vi "Read Test Data (DC Parallel Total Manual Mode).vi"(0 "VISA resource name":refnum<visa-resource-name>, 11 "error in (no error)":errorcluster) -> (4 "VISA resource name out":refnum<visa-resource-name>, 6 "Test Meter Data Output":T1 {"Voltage (V)" format="%.1f"; "RMS Current (A)" format="%.3f"; "Power (W)" format="%.1f"}, 15 "error out":errorcluster)   [LabVIEW 2016, in "APT 300XAC Series.lvlib"]
doc: "Reads the DC mode <B>active data being displayed on the LCD display</B> while the test is in process. It also gives the last data taken when the test sequence compled. \n\nIn DC Mode the output data cluster has the following data.\n\n1. Memory\n2. Timer (s)\n3. Voltage (V)\n4. RMS Current (A)\n5. Power (W)\n6. Status"
uses:
  APT 300XAC Series.lvlib
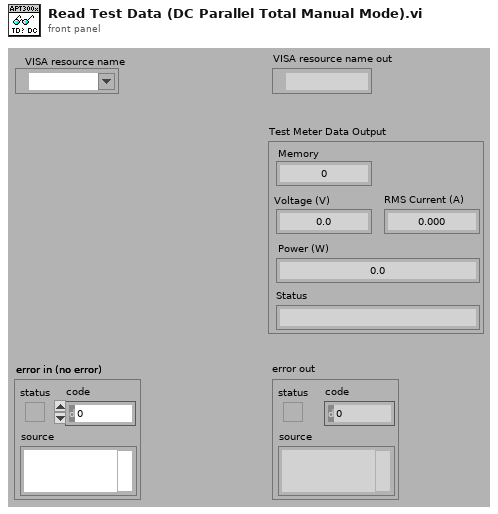
[diagram p1: front panel]
types:
  T1 = cluster{"Memory":dbl, "Voltage (V)":dbl, "RMS Current (A)":dbl, "Power (W)":dbl, "Status":string}
  T2 = cluster{"Memory":i32, "Volt":dbl, "Current":dbl, "Power":dbl, "Status":string}
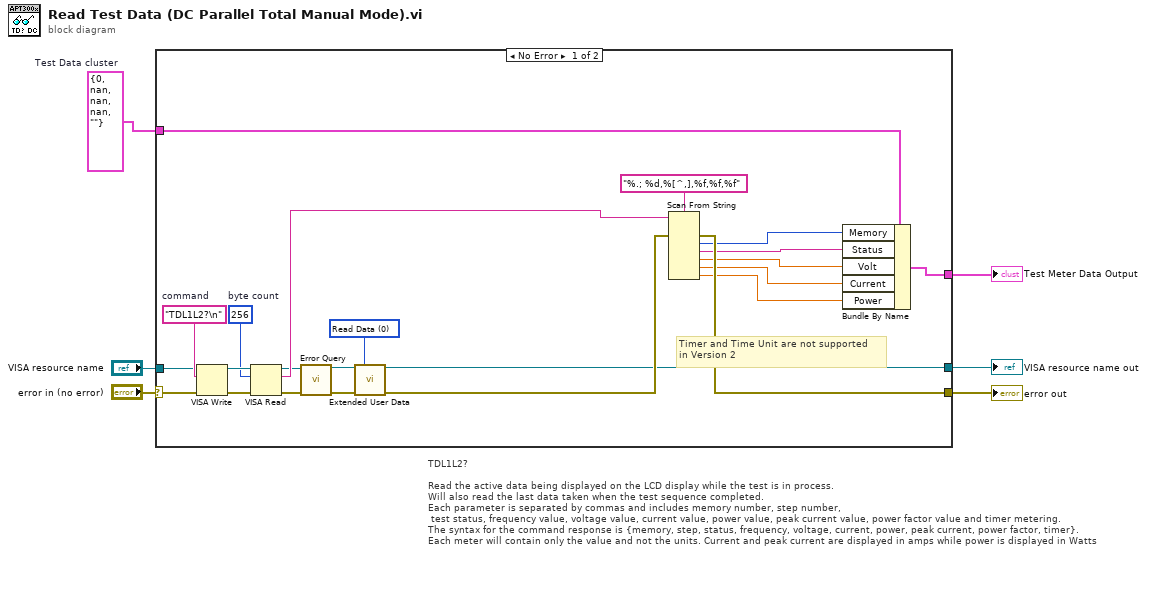
[diagram p0: block diagram]
diagram:
  w2 = T2 {"Memory"=0, "Volt"=nan, "Current"=nan, "Power"=nan, "Status"=""}  # Test Data cluster
  # "TDL1L2?\n\nRead the active data being displayed on the LCD display while the test is in process. \nWill also read the last data taken when the test sequence completed. \nEach parameter is separated by commas and includes memory number, step number,\n test status, frequency value, voltage value, current value, power value, peak current value, power factor value and timer metering. \nThe syntax for the command response is {memory, step, status, frequency, voltage, current, power, peak current, power factor, timer}. \nEach meter will contain only the value and not the units. Current and peak current are displayed in amps while power is displayed in Watts"
  n1 = case shown="No Error" "error in (no error)" {
    selector: "error in (no error)" -> [w22 w31]
    tunnel: "VISA resource name" -> [w23 w32]
    tunnel: [w13 w32] -> w4
    tunnel: [w21 w31] -> w3
    tunnel: [w26 w30] -> w1
    tunnel: w2 -> [w25 w30]
    frame No Error {
      w17 = u16 0 items=["Read Data", "Write Data", "Clear Data", "Clear ALL Data"] ("Action")
      w24 = "TDL1L2?\n"  # command
      w27 = u32 256  # byte count
      # "Timer and Time Unit are not supported\nin Version 2"
      n2 = VISA Write(VISA resource name=w23, write buffer=w24, error in (no error)=w22) -> (VISA resource name out=w29:refnum<visa-resource-name>, error out=w28:errorcluster)  [unwired: 1 out]
      n3 = VISA Read(VISA resource name=w29, byte count=w27, error in (no error)=w28) -> (VISA resource name out=w19:refnum<visa-resource-name>, read buffer=w20:string, error out=w18:errorcluster)  [unwired: 1 out]
      n4 = call "Error Query.vi"("VISA resource name"=w19, "error in (no error)"=w18) -> ("VISA resource name out"=w14:refnum<visa-resource-name>, "error out"=w15:errorcluster)  [unwired: 10 in, 2 out]
      n5 = call "Extended User Data.vi"("VISA resource name"=w14, "Action"=w17, "Error In (no error)"=w15) -> ("VISA resource name out"=w13:refnum<visa-resource-name>, "Error Out"=w16:errorcluster)  [unwired: 10 in, 1 out]
      n6 = Scan From String(format string="%.; %d,%[^,],%f,%f,%f", input string=w20, error in=w16) -> (error out=w21:errorcluster, output 1=w11:i32, output 2=w10:string, output 3=w9:dbl, output 4=w8:dbl, output 5=w7:dbl)  [unwired: 6 in, 2 out]
      n7 = Bundle By Name(cluster=w25, "Memory"=w11, "Status"=w10, "Volt"=w9, "Current"=w8, "Power"=w7) -> (w26:T2)
    }
    frame Error {
    }
  }
  "VISA resource name out" <- w4
  "error out" <- w3
  "Test Meter Data Output" <- w1
